vi "Get Auxiliary Amplifier Mode.vi"(8 "error in (no error)":errorcluster, 11 "VISA resource name":refnum<visa-resource-name>) -> (0 "error out":errorcluster, 2 "Amplifier Mode":u16, 3 "VISA resource name out":refnum<visa-resource-name>)   [LabVIEW 2011, in "Fluke 5XXX Series Multicalibrators.lvlib"]
doc: "This VI returns state of the auxiliary amplifier if the auxiliary amplifier is present in the system.\n\nNotes:\n\n(1) Instrument model 5520A and 57LFC can not use auxiliary amplifier."
uses:
  Fluke 5XXX Series Multicalibrators.lvlib
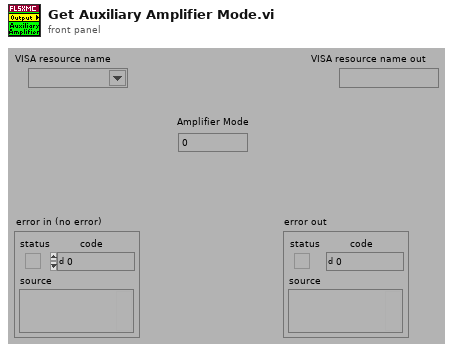
[diagram p1: front panel]
types:
  T1 = cluster{"Status":bool, "Code":i32, "Source (VI Name)":string}
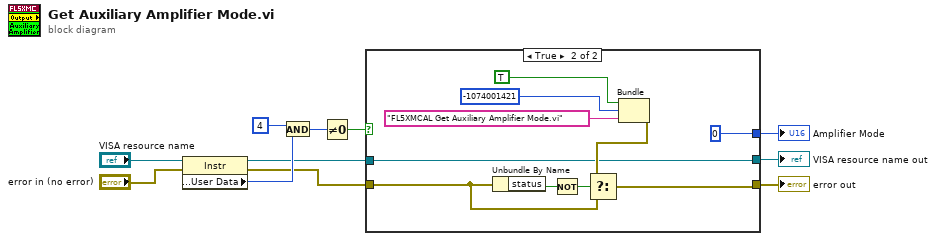
[diagram p0: block diagram]
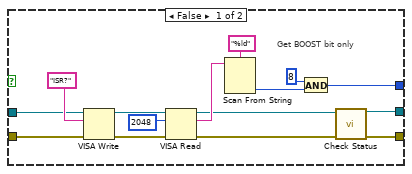
[diagram p2: hidden frame]
diagram:
  n1 = property class="Instr"(reference="VISA resource name", error in="error in (no error)") -> (reference out=w3:refnum<visa-resource-name>, error out=w2:errorcluster, "General Settings:User Data"=w8:u32)
  n2 = And(x=4 ("Numeric"), y=w8) -> (x .and. y?=w7:u32)
  n3 = Not Equal To 0?(x=w7) -> (x != 0?=w1:bool)
  n4 = case shown="True" w1 {
    tunnel: [w17 w27] -> w10
    tunnel: [w14 w28] -> w9
    tunnel: [w18 0] -> w11
    tunnel: w3 -> [w13 w28]
    tunnel: w2 -> [w12 w29]
    frame False {
      # "Get BOOST bit only"
      n5 = VISA Write(VISA resource name=w13, write buffer="ISR?", error in (no error)=w12) -> (VISA resource name out=w25:refnum<visa-resource-name>, error out=w24:errorcluster)  [unwired: 1 out]
      n6 = VISA Read(VISA resource name=w25, byte count=u32 2048 ("byte count (0)"), error in (no error)=w24) -> (VISA resource name out=w15:refnum<visa-resource-name>, read buffer=w21:string, error out=w16:errorcluster)  [unwired: 1 out]
      n7 = Scan From String(format string="%ld", input string=w21) -> (output 1=w19:i32)  [unwired: 3 in, 3 out]
      n8 = And(x=8, y=w19) -> (x .and. y?=w18:i32)
      n9 = call "Check Status.vi"("VISA resource name"=w15, "error in (no error)"=w16) -> ("VISA resource name out"=w14:refnum<visa-resource-name>, "error out"=w17:errorcluster)  [unwired: 12 in]
    }
    frame True {
      n10 = Unbundle By Name(w29) -> ("status"=w32:bool)
      n11 = Not(x=w32) -> (.not. x?=w31:bool)
      n12 = Bundle("Status"=TRUE, "Code"=-1074001421, "Source (VI Name)"="FL5XMCAL Get Auxiliary Amplifier Mode.vi") -> (w30:T1)  [unwired: 1 in]
      n13 = Select(t=w30, s=w31, f=w29) -> (s? t:f=w27:errorcluster)
    }
  }
  "Amplifier Mode" <- w11
  "VISA resource name out" <- w9
  "error out" <- w10
